vi "GetActiveFrame.vi"(6 "error in":errorcluster, 9 "DiagramDisable in":refnum<class "DiagramDisable.lvclass">) -> (0 "error out":errorcluster, 3 "DiagramDisable out":refnum<class "DiagramDisable.lvclass">)   [LabVIEW 2014, in "DiagramDisable.lvclass"]
uses:
  DiagramDisable.lvclass
  DiagramDisable.lvclass/DiagramDisable.ctl
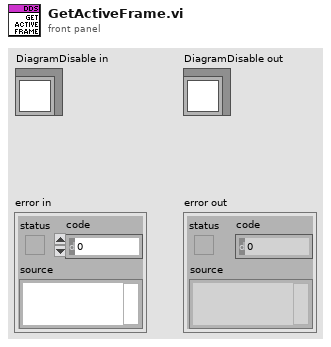
[diagram p1: front panel]
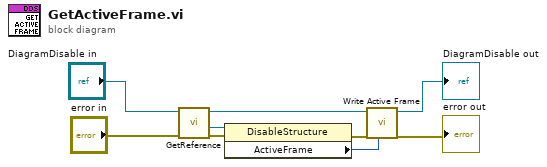
[diagram p0: block diagram]
diagram:
  n1 = call "GetReference.vi"("error in"="error in", "DiagramDisable in"="DiagramDisable in") -> ("error out"=w6:errorcluster, "DDS reference"=w7:refnum<vi>, "DiagramDisable out"=w2:refnum<class "DiagramDisable.lvclass">)  [unwired: 7 in]
  n2 = property class="DisableStructure"(reference=w7, error in=w6) -> (error out=→"error out":errorcluster, "ActiveFrame"=w3:i16)  [unwired: 1 out]
  n3 = call "Write Active Frame.vi"("Active Frame"=w3, "DiagramDisable in"=w2) -> ("DiagramDisable out"=→"DiagramDisable out":refnum<class "DiagramDisable.lvclass">)  [unwired: 7 in]
